vi "roller_user_state_store.vi"(10 "data_store_mode":enum16{"Set", "Get"}(ring), 11 "roller user state":T1) -> (3 "roller user state out":T1)   [LabVIEW 2011]
uses:
  roller_user_state.ctl
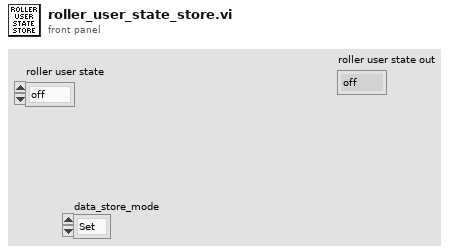
[diagram p1: front panel]
types:
  T1 = typedef "roller_user_state.ctl" = enum16{"off", "collect", "blow", "force suck"}
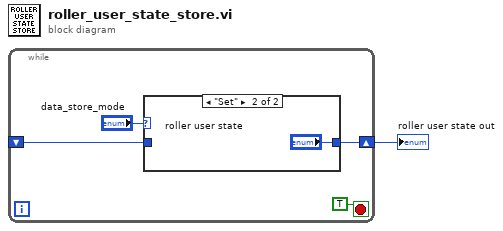
[diagram p0: block diagram]
diagram:
  n1 = while {
    shift-right: [w3] -> w1
    shift-left: _ -> [w2]
    stop <- TRUE stop-if-true
    n2 = case shown="\"Set\"" "data_store_mode" {
      tunnel: [w6 "roller user state"] -> w3
      tunnel: w2 -> [w6 _]
      frame "Get", Default {
      }
      frame "Set" {
      }
    }
  }
  "roller user state out" <- w1
